vi "Windows GUI.vi"() -> ()   [LabVIEW 2023]
doc: "This example is based on NI's basic Producer/Consumer template and shows how a WebSocket client can communicate with a REST server that handles upgrading HTTP connections to WebSockets.\n\nUses a helper VIG to manage the actual WebSocket object including sending/receiving messages."
uses:
  WebSocket/Stats.ctl
  WebSocket VIG States.ctl
  WebSocket/WebSocket.lvclass
panel:
  out "TxStats":T1
  out "RxStats":T1
  out "Latest Sample":dbl
  in  "Phase":dbl
  in  "Frequency":dbl=1.0
  in  "Amplitude":dbl=1.0
  out "Waveform Graph":dbl[](graph)
  out "Connected?":bool
  in  "Connect":bool
  in  "RT IP":string="192.168.0.118"
  in  "stop":bool
  # "To RT"
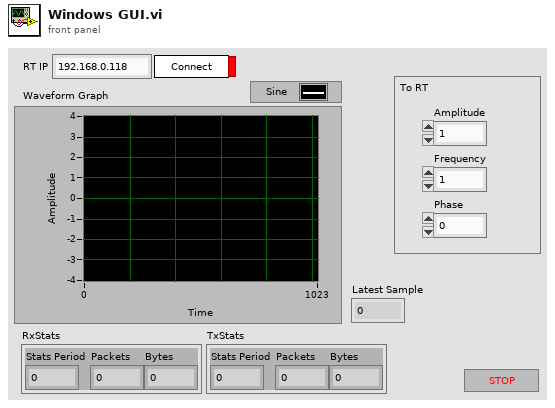
[diagram p1: front panel]
types:
  T1 = typedef "WebSocket.lvclass/Stats.ctl" = cluster{"Stats Period":dbl, "Packets":u64, "Bytes":u64}
  T2 = typedef "WebSocket VIG States.ctl" = enum16{"Open", "Close", "Send", "Receive", "Check"}
  T3 = cluster{"type":string, "tag":string, "value":dbl}
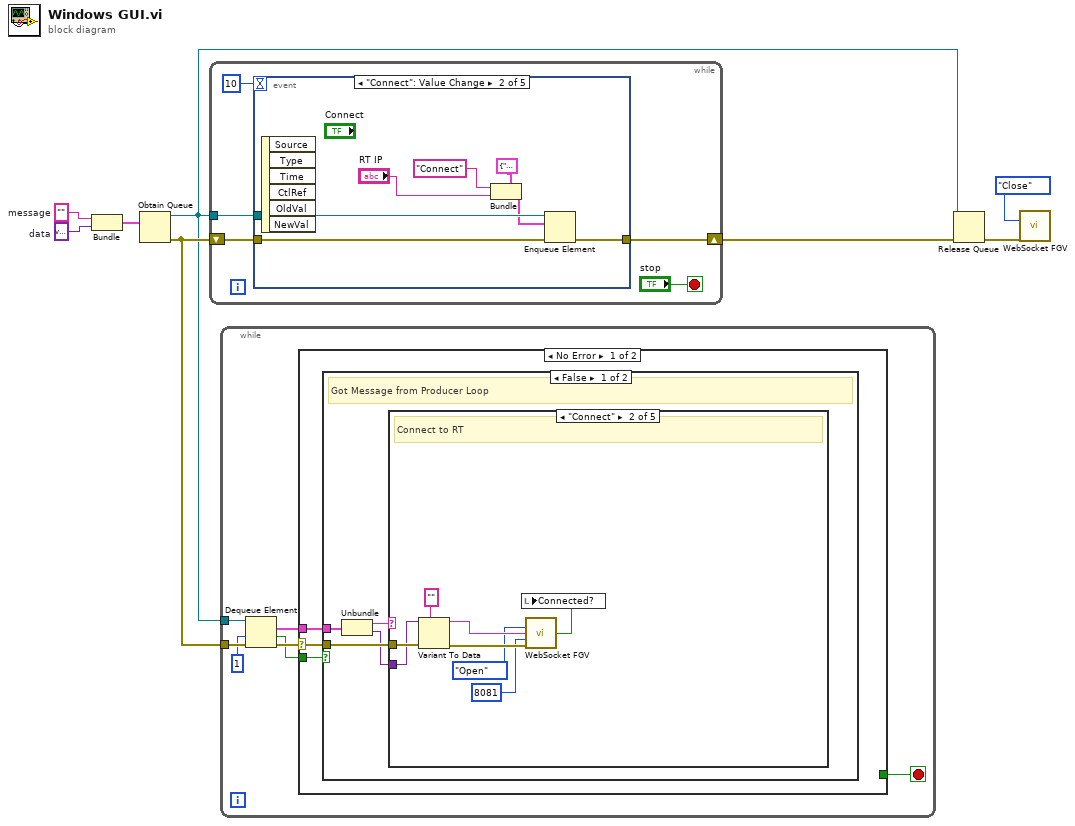
[diagram p0: block diagram]
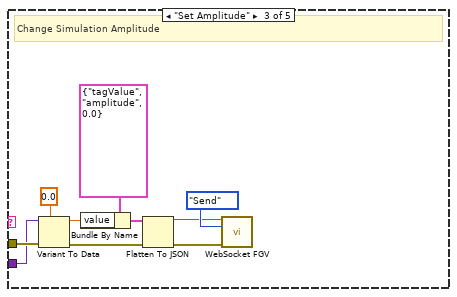
[diagram p3: hidden frame]
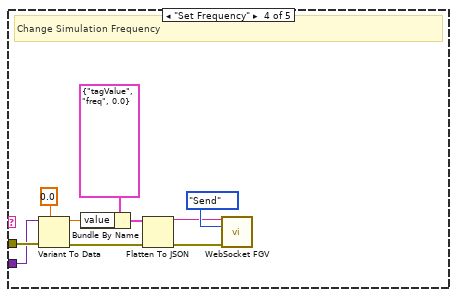
[diagram p4: hidden frame]
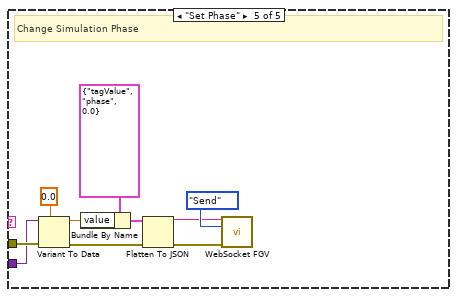
[diagram p5: hidden frame]
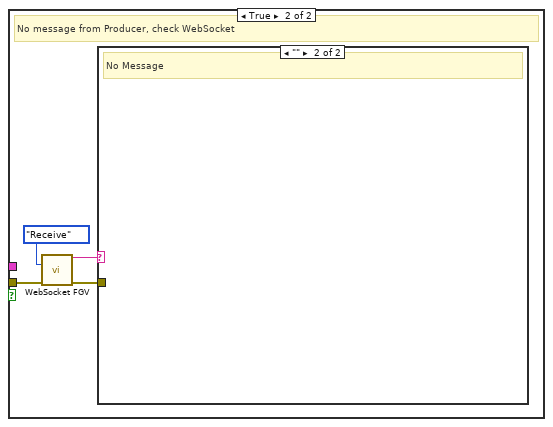
[diagram p6: hidden frame]
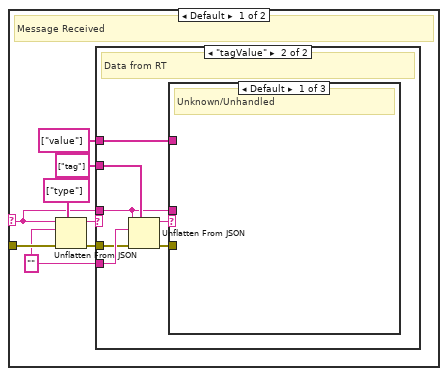
[diagram p7: hidden frame]
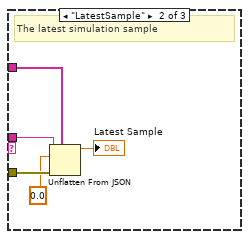
[diagram p9: hidden frame]
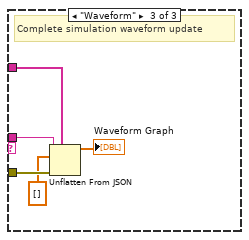
[diagram p10: hidden frame]
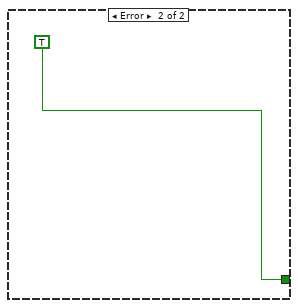
[diagram p11: hidden frame]
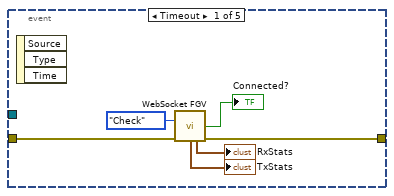
[diagram p12: hidden frame]
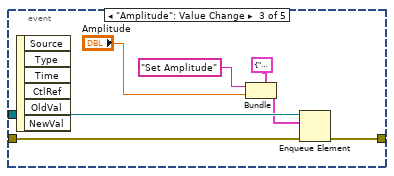
[diagram p13: hidden frame]
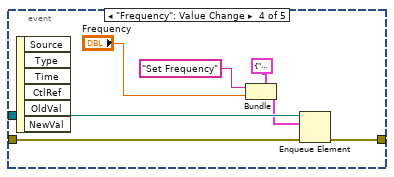
[diagram p14: hidden frame]
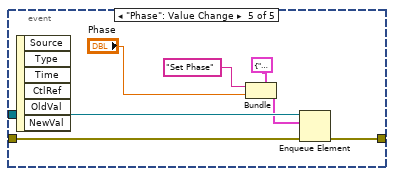
[diagram p15: hidden frame]
diagram:
  w5 = variant  # data
  w6 = ""  # message
  n1 = Bundle("message"=w6, "data"=w5) -> (w7:cluster{"message":string, "data":variant})  [unwired: 1 in]
  n2 = Obtain Queue(element data type=w7) -> (queue out=w3:refnum<queue>, error out=w4:errorcluster)  [unwired: 4 in, 1 out]
  n3 = while {
    shift-right: [w10] -> w8
    shift-left: w4 -> [w12]
    tunnel: w3 -> [w11]
    stop <- "stop" stop-if-true
    n4 = event shown="[1] \"Connect\": Value Change" {
      selector: _ -> [_ _ _ _ _]
      dyn-events: _ -> [_ _ _ _ _]
      timeout: 10 -> [_ _ _ _ _]
      tunnel: w12 -> [w18 w25 w32 w39 w46]
      tunnel: w11 -> [_ w24 w31 w38 w45]
      tunnel: [w19 w26 w33 w40 w47] -> w10
      event Timeout {
        n5 = event-data() -> ()  [unwired: 1 in, 3 out]
        n6 = call "WebSocket FGV.vi"("Action"=WebSocket_VIG_States."Check", "error in (no error)"=w18) -> ("Connection Status"=→"Connected?":bool, "TxStats"=→"TxStats":T1, "RxStats"=→"RxStats":T1, "error out"=w19:errorcluster)  [unwired: 8 in, 2 out]
      }
      event "Connect": Value Change {
        n7 = event-data() -> ()  [unwired: 1 in, 6 out]
        n8 = Bundle(cluster=cluster{"message":string, "data":variant} {"message"="", "data"=variant} ("element"), "message"="Connect", "data"="RT IP") -> (w22:cluster{"message":string, "data":variant})
        n9 = Enqueue Element(queue=w24, element=w22, error in (no error)=w25) -> (error out=w26:errorcluster)  [unwired: 1 in, 2 out]
      }
      event "Amplitude": Value Change {
        n10 = event-data() -> ()  [unwired: 1 in, 6 out]
        n11 = Bundle(cluster=cluster{"message":string, "data":variant} {"message"="", "data"=variant} ("element"), "message"="Set Amplitude", "data"="Amplitude") -> (w29:cluster{"message":string, "data":variant})
        n12 = Enqueue Element(queue=w31, element=w29, error in (no error)=w32) -> (error out=w33:errorcluster)  [unwired: 1 in, 2 out]
      }
      event "Frequency": Value Change {
        n13 = event-data() -> ()  [unwired: 1 in, 6 out]
        n14 = Bundle(cluster=cluster{"message":string, "data":variant} {"message"="", "data"=variant} ("element"), "message"="Set Frequency", "data"="Frequency") -> (w36:cluster{"message":string, "data":variant})
        n15 = Enqueue Element(queue=w38, element=w36, error in (no error)=w39) -> (error out=w40:errorcluster)  [unwired: 1 in, 2 out]
      }
      event "Phase": Value Change {
        n16 = event-data() -> ()  [unwired: 1 in, 6 out]
        n17 = Bundle(cluster=cluster{"message":string, "data":variant} {"message"="", "data"=variant} ("element"), "message"="Set Phase", "data"="Phase") -> (w43:cluster{"message":string, "data":variant})
        n18 = Enqueue Element(queue=w45, element=w43, error in (no error)=w46) -> (error out=w47:errorcluster)  [unwired: 1 in, 2 out]
      }
    }
  }
  n19 = while {
    tunnel: w3 -> [w54]
    tunnel: w4 -> [w50]
    stop <- w51 stop-if-true
    n20 = Dequeue Element(queue=w54, timeout in ms (-1)=1, error in (no error)=w50) -> (element=w52:cluster{"message":string, "data":variant}, timed out?=w49:bool, error out=w53:errorcluster)  [unwired: 1 out]
    n21 = case shown="No Error" w53 {
      selector: w53 -> [w55 _]
      tunnel: w52 -> [w56 _]
      tunnel: [_ TRUE] -> w51
      tunnel: w49 -> [w57 _]
      frame No Error {
        n22 = case shown="False" w57 {
          tunnel: w56 -> [w61 _]
          tunnel: w55 -> [w59 w103]
          frame False {
            # "Got Message from Producer Loop"
            n23 = Unbundle(w61) -> ("message"=w60:string, "data"=w58:variant)
            n24 = case shown="\"Connect\"" w60 {
              tunnel: w59 -> [_ w69 w79 w89 w99]
              tunnel: w58 -> [_ w68 w78 w88 w98]
              frame Default {
                # "Unknown/Unhandled"
              }
              frame "Connect" {
                # "Connect to RT"
                n25 = Variant To Data(error in=w69, type="", Variant=w68) -> (data=w65:string, error out=w66:errorcluster)
                n26 = call "WebSocket FGV.vi"("Action"=WebSocket_VIG_States."Open", "TCP Address"=w65, "TCP Port"=u32 8081, "error in (no error)"=w66) -> ("Connection Status"=w62:bool)  [unwired: 6 in, 5 out]
                n27 = local write "Connected?"(w62) -> ()
              }
              frame "Set Amplitude" {
                # "Change Simulation Amplitude"
                n28 = Variant To Data(error in=w79, type=0.0, Variant=w78) -> (data=w73:dbl, error out=w76:errorcluster)
                n29 = Bundle By Name(cluster=T3 {"type"="tagValue", "tag"="amplitude", "value"=0.0}, "value"=w73) -> (w71:T3)
                n30 = Flatten To JSON(anything=w71, error in (no error)=w76) -> (JSON string=w70:string, 11:w72:errorcluster)  [unwired: 1 in]
                n31 = call "WebSocket FGV.vi"("Tx to Server"=w70, "Action"=WebSocket_VIG_States."Send", "error in (no error)"=w72) -> ()  [unwired: 7 in, 6 out]
              }
              frame "Set Frequency" {
                # "Change Simulation Frequency"
                n32 = Variant To Data(error in=w89, type=0.0, Variant=w88) -> (data=w83:dbl, error out=w86:errorcluster)
                n33 = Bundle By Name(cluster=T3 {"type"="tagValue", "tag"="freq", "value"=0.0}, "value"=w83) -> (w81:T3)
                n34 = Flatten To JSON(anything=w81, error in (no error)=w86) -> (JSON string=w80:string, 11:w82:errorcluster)  [unwired: 1 in]
                n35 = call "WebSocket FGV.vi"("Tx to Server"=w80, "Action"=WebSocket_VIG_States."Send", "error in (no error)"=w82) -> ()  [unwired: 7 in, 6 out]
              }
              frame "Set Phase" {
                # "Change Simulation Phase"
                n36 = Variant To Data(error in=w99, type=0.0, Variant=w98) -> (data=w93:dbl, error out=w96:errorcluster)
                n37 = Bundle By Name(cluster=T3 {"type"="tagValue", "tag"="phase", "value"=0.0}, "value"=w93) -> (w91:T3)
                n38 = Flatten To JSON(anything=w91, error in (no error)=w96) -> (JSON string=w90:string, 11:w92:errorcluster)  [unwired: 1 in]
                n39 = call "WebSocket FGV.vi"("Tx to Server"=w90, "Action"=WebSocket_VIG_States."Send", "error in (no error)"=w92) -> ()  [unwired: 7 in, 6 out]
              }
            }
          }
          frame True {
            # "No message from Producer, check WebSocket"
            n40 = call "WebSocket FGV.vi"("Action"=WebSocket_VIG_States."Receive", "error in (no error)"=w103) -> ("Rx from Server"=w101:string, "error out"=w100:errorcluster)  [unwired: 8 in, 4 out]
            n41 = case shown="\"\"" w101 {
              selector: w101 -> [w105 _]
              tunnel: w100 -> [w110 _]
              frame Default {
                w104 = ""
                # "Message Received"
                n42 = Unflatten From JSON(path=string[] ["type"], JSON string=w105, type and defaults=w104, error in (no error)=w110) -> (value=w108:string, error out=w109:errorcluster)  [unwired: 3 in]
                n43 = case shown="\"tagValue\"" w108 {
                  tunnel: w109 -> [_ w117]
                  tunnel: string[] ["tag"] -> [_ w116]
                  tunnel: string[] ["value"] -> [_ w112]
                  tunnel: w105 -> [_ w113]
                  tunnel: w104 -> [_ w118]
                  frame Default {
                    # "Unhandled Packet Type"
                  }
                  frame "tagValue" {
                    # "Data from RT"
                    n44 = Unflatten From JSON(path=w116, JSON string=w113, type and defaults=w118, error in (no error)=w117) -> (value=w114:string, error out=w115:errorcluster)  [unwired: 3 in]
                    n45 = case shown="Default" w114 {
                      tunnel: w115 -> [_ w121 w126]
                      tunnel: w113 -> [_ w123 w128]
                      tunnel: w112 -> [_ w122 w127]
                      frame Default {
                        # "Unknown/Unhandled"
                      }
                      frame "LatestSample" {
                        # "The latest simulation sample"
                        n46 = Unflatten From JSON(path=w122, JSON string=w123, type and defaults=0.0, error in (no error)=w121) -> (value=→"Latest Sample":dbl)  [unwired: 3 in, 1 out]
                      }
                      frame "Waveform" {
                        # "Complete simulation waveform update"
                        n47 = Unflatten From JSON(path=w127, JSON string=w128, type and defaults=dbl[] [], error in (no error)=w126) -> (value=→"Waveform Graph":dbl[])  [unwired: 3 in, 1 out]
                      }
                    }
                  }
                }
              }
              frame "" {
                # "No Message"
              }
            }
          }
        }
      }
      frame Error {
      }
    }
  }
  n48 = Release Queue(queue=w3, error in (no error)=w8) -> (error out=w2:errorcluster)  [unwired: 1 in, 2 out]
  n49 = call "WebSocket FGV.vi"("Action"=WebSocket_VIG_States."Close", "error in (no error)"=w2) -> ()  [unwired: 8 in, 6 out]
